vi "Create Lookup Table Envelope Waveform.vi"(0 "Reference Waveform":T2 {"Runtime Scaling" format="%#_6p"; "Sample Rate" format="%#_6p"; "Burst Length (s)" format="%#_6p"; "PAPR (dB)" format="%.2f"; "Signal Bandwidth (Hz)" format="%#_6p"}, 5 "Lookup Table Configuration":T1={"Supply Voltage (V)"=array[1024 elements], "DUT Input Power (dBm)"=array[1024 elements]}, 11 "error in (no error)":errorcluster) -> (4 "Detrough Envelope Waveform":T2 {"Runtime Scaling" format="%#_6p"; "Sample Rate" format="%#_6p"; "Burst Length (s)" format="%#_6p"; "PAPR (dB)" format="%.2f"; "Signal Bandwidth (Hz)" format="%#_6p"}, 15 "error out":errorcluster)   [LabVIEW 2016, in "Envelope Tracking.lvlib"]
uses:
  Envelope Tracking.lvlib
  Common/Waveform.ctl
  Typedefs/Lookup Table Configuration.ctl
  Common/Common.lvlib
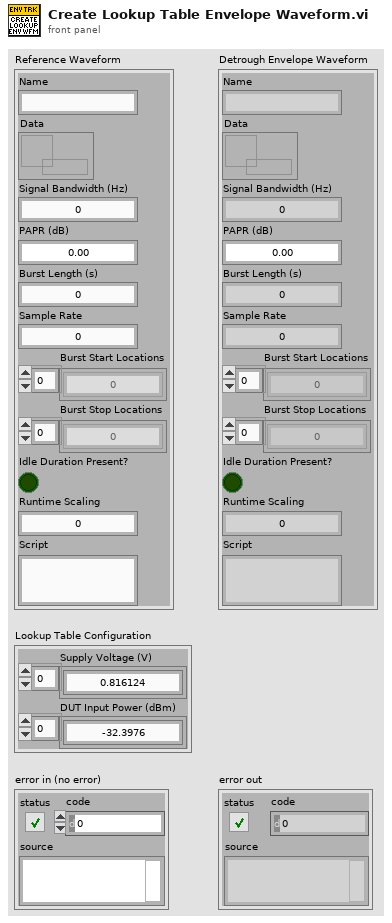
[diagram p1: front panel]
types:
  T1 = typedef "Envelope Tracking.lvlib/Lookup Table Configuration.ctl" = cluster{"Supply Voltage (V)":sgl[], "DUT Input Power (dBm)":sgl[]}
  T2 = typedef "Common.lvlib/Waveform.ctl" = cluster{"Name":string, "Data":refnum<data-value>, "Signal Bandwidth (Hz)":dbl, "PAPR (dB)":dbl, "Burst Length (s)":dbl, "Sample Rate":dbl, "Burst Start Locations":i32[], "Burst Stop Locations":i32[], "Idle Duration Present?":bool, "Runtime Scaling":dbl, "Script":string}
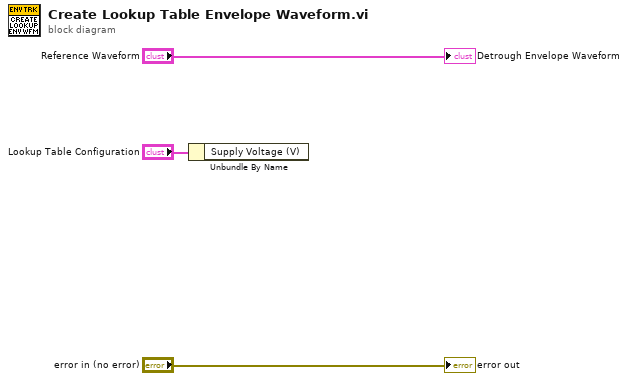
[diagram p0: block diagram]
diagram:
  n1 = Unbundle By Name("Lookup Table Configuration") -> ()  [unwired: 1 out]
  "Detrough Envelope Waveform" <- "Reference Waveform"
  "error out" <- "error in (no error)"
